vi "GeoData.vi"() -> ()   [LabVIEW 2017] (continued)
County\tH4\n6098\t9005\tWinsted\tCT\tLitchfield County\tH4\n6763\t9005\tMorris\tCT\tLitchfield County\tH4\n6779\t9005\tOakville\tCT\tLitchfield County\tH4\n6793\t9005\tWashington\tCT\tLitchfield County\tH4\n6786\t9005\tTerryville\tCT\tLitchfield County\tH4\n6782\t9005\tPlymouth\tCT\tLitchfield County\tH4\n6759\t9005\tLitchfield\tCT\tLitchfield County\tH4\n6753\t9005\tCornwall\tCT\tLitchfield County\tH4\n6708\t9005\tWaterbury\tCT\tLitchfield County\tH4\n6750\t9005\tBantam\tCT\tLitchfield County\tH4\n6756\t9005\tGoshen\tCT\tLitchfield County\tH4\n6757\t9005\tKent\tCT\tLitchfield County\tH4\n6068\t9005\tSalisbury\tCT\tLitchfield County\tH4\n6755\t9005\tGaylordsville\tCT\tLitchfield County\tH4\n6781\t9005\tPequabuck\tCT\tLitchfield County\tH4\n6792\t9005\tTorrington\tCT\tLitchfield County\tH4\n6031\t9005\tFalls village\tCT\tLitchfield County\tH4\n6069\t9005\tSharon\tCT\tLitchfield County\tH4\n6063\t9005\tBarkhamsted\tCT\tLitchfield County\tH4\n6751\t9005\tBethlehem\tCT\tLitchfield County\tH4\n6784\t9005\tSherman\tCT\tLitchfield County\tH4\n6791\t9005\tHarwinton\tCT\tLitchfield County\tH4\n6794\t9005\tWashington depot\tCT\tLitchfield County\tH4\n6804\t9005\tBrookfield\tCT\tLitchfield County\tH4\n6065\t9005\tRiverton\tCT\tLitchfield County\tH4\n6785\t9005\tSouth kent\tCT\tLitchfield County\tH4\n6783\t9005\tRoxbury\tCT\tLitchfield County\tH4\n6059\t9005\tNorth canton\tCT\tLitchfield County\tH4\n6010\t9005\tBristol\tCT\tLitchfield County\tH4\n6790\t9005\tTorrington\tCT\tLitchfield County\tH4\n6018\t9005\tCanaan\tCT\tLitchfield County\tH4\n6777\t9005\tNew preston marble dale\tCT\tLitchfield County\tH4\n6776\t9005\tNew milford\tCT\tLitchfield County\tH4\n6752\t9005\tBridgewater\tCT\tLitchfield County\tH4\n6796\t9005\tWest cornwall\tCT\tLitchfield County\tH4\n6079\t9005\tTaconic\tCT\tLitchfield County\tH4\n6024\t9005\tEast canaan\tCT\tLitchfield County\tH4\n6061\t9005\tPine meadow\tCT\tLitchfield County\tH4\n6039\t9005\tLakeville\tCT\tLitchfield County\tH4\n6058\t9005\tNorfolk\tCT\tLitchfield County\tH4\n6778\t9005\tNorthfield\tCT\tLitchfield County\tH4\n6798\t9005\tWoodbury\tCT\tLitchfield County\tH4\n6795\t9005\tWatertown\tCT\tLitchfield County\tH4\n6787\t9005\tThomaston\tCT\tLitchfield County\tH4\n6754\t9005\tCornwall bridge\tCT\tLitchfield County\tH4\n6758\t9005\tLakeside\tCT\tLitchfield County\tH4\n6073\t9007\tSouth glastonbury\tCT\tMiddlesex County\tH4\n6413\t9007\tClinton\tCT\tMiddlesex County\tH4\n6422\t9007\tDurham\tCT\tMiddlesex County\tH4\n6424\t9007\tEast hampton\tCT\tMiddlesex County\tH4\n6441\t9007\tHigganum\tCT\tMiddlesex County\tH4\n6420\t9007\tSalem\tCT\tMiddlesex County\tH4\n6442\t9007\tIvoryton\tCT\tMiddlesex County\tH4\n6456\t9007\tMiddle haddam\tCT\tMiddlesex County\tH4\n6426\t9007\tEssex\tCT\tMiddlesex County\tH4\n6475\t9007\tOld saybrook\tCT\tMiddlesex County\tH4\n6023\t9007\tEast berlin\tCT\tMiddlesex County\tH4\n6469\t9007\tMoodus\tCT\tMiddlesex County\tH4\n6480\t9007\tPortland\tCT\tMiddlesex County\tH4\n6414\t9007\tCobalt\tCT\tMiddlesex County\tH4\n6423\t9007\tEast haddam\tCT\tMiddlesex County\tH4\n6416\t9007\tCromwell\tCT\tMiddlesex County\tH4\n6409\t9007\tCenterbrook\tCT\tMiddlesex County\tH4\n6457\t9007\tMiddletown\tCT\tMiddlesex County\tH4\n6455\t9007\tMiddlefield\tCT\tMiddlesex County\tH4\n6459\t9007\tMiddletown\tCT\tMiddlesex County\tH4\n6412\t9007\tChester\tCT\tMiddlesex County\tH4\n6415\t9007\tColchester\tCT\tMiddlesex County\tH4\n6417\t9007\tDeep river\tCT\tMiddlesex County\tH4\n6419\t9007\tKillingworth\tCT\tMiddlesex County\tH4\n6438\t9007\tHaddam\tCT\tMiddlesex County\tH4\n6498\t9007\tWestbrook\tCT\tMiddlesex County\tH4\n6481\t9007\tRockfall\tCT\tMiddlesex County\tH4\n6422\t9009\tDurham\tCT\tNew Haven County\tH4\n6403\t9009\tBeacon falls\tCT\tNew Haven County\tH4\n6450\t9009\tMeriden\tCT\tNew Haven County\tH4\n6443\t9009\tMadison\tCT\tNew Haven County\tH4\n6483\t9009\tSeymour\tCT\tNew Haven County\tH4\n6770\t9009\tNaugatuck\tCT\tNew Haven County\tH4\n6779\t9009\tOakville\tCT\tNew Haven County\tH4\n6521\t9009\tNew haven\tCT\tNew Haven County\tH4\n6493\t9009\tWallingford\tCT\tNew Haven County\tH4\n6509\t9009\tNew haven\tCT\tNew Haven County\tH4\n6501\t9009\tNew haven\tCT\tNew Haven County\tH4\n6749\t9009\tWaterbury\tCT\tNew Haven County\tH4\n6703\t9009\tWaterbury\tCT\tNew Haven County\tH4\n6401\t9009\tAnsonia\tCT\tNew Haven County\tH4\n6461\t9009\tMilford\tCT\tNew Haven County\tH4\n6460\t9009\tMilford\tCT\tNew Haven County\tH4\n6489\t9009\tSouthington\tCT\tNew Haven County\tH4\n6511\t9009\tNew haven\tCT\tNew Haven County\tH4\n6720\t9009\tWaterbury\tCT\tNew Haven County\tH4\n6724\t9009\tWaterbury\tCT\tNew Haven County\tH4\n6533\t9009\tNew haven\tCT\tNew Haven County\tH4\n6488\t9009\tSouthbury\tCT\tNew Haven County\tH4\n6516\t9009\tWest haven\tCT\tNew Haven County\tH4\n6517\t9009\tHamden\tCT\tNew Haven County\tH4\n6518\t9009\tHamden\tCT\tNew Haven County\tH4\n6520\t9009\tNew haven\tCT\tNew Haven County\tH4\n6524\t9009\tBethany\tCT\tNew Haven County\tH4\n6708\t9009\tWaterbury\tCT\tNew Haven County\tH4\n6410\t9009\tCheshire\tCT\tNew Haven County\tH4\n6702\t9009\tWaterbury\tCT\tNew Haven County\tH4\n6532\t9009\tNew haven\tCT\tNew Haven County\tH4\n6505\t9009\tNew haven\tCT\tNew Haven County\tH4\n6507\t9009\tNew haven\tCT\tNew Haven County\tH4\n6411\t9009\tCheshire\tCT\tNew Haven County\tH4\n6037\t9009\tBerlin\tCT\tNew Haven County\tH4\n6418\t9009\tDerby\tCT\tNew Haven County\tH4\n6451\t9009\tMeriden\tCT\tNew Haven County\tH4\n6473\t9009\tNorth haven\tCT\tNew Haven County\tH4\n6477\t9009\tOrange\tCT\tNew Haven County\tH4\n6514\t9009\tHamden\tCT\tNew Haven County\tH4\n6510\t9009\tNew haven\tCT\tNew Haven County\tH4\n6515\t9009\tNew haven\tCT\tNew Haven County\tH4\n6762\t9009\tMiddlebury\tCT\tNew Haven County\tH4\n6487\t9009\tSouth britain\tCT\tNew Haven County\tH4\n6723\t9009\tWaterbury\tCT\tNew Haven County\tH4\n6701\t9009\tWaterbury\tCT\tNew Haven County\tH4\n6530\t9009\tNew haven\tCT\tNew Haven County\tH4\n6495\t9009\tWallingford\tCT\tNew Haven County\tH4\n6504\t9009\tNew haven\tCT\tNew Haven County\tH4\n6535\t9009\tNew haven\tCT\tNew Haven County\tH4\n6536\t9009\tNew haven\tCT\tNew Haven County\tH4\n6437\t9009\tGuilford\tCT\tNew Haven County\tH4\n6492\t9009\tWallingford\tCT\tNew Haven County\tH4\n6479\t9009\tPlantsville\tCT\tNew Haven County\tH4\n6471\t9009\tNorth branford\tCT\tNew Haven County\tH4\n6525\t9009\tWoodbridge\tCT\tNew Haven County\tH4\n6706\t9009\tWaterbury\tCT\tNew Haven County\tH4\n6712\t9009\tProspect\tCT\tNew Haven County\tH4\n6506\t9009\tNew haven\tCT\tNew Haven County\tH4\n6502\t9009\tNew haven\tCT\tNew Haven County\tH4\n6534\t9009\tNew haven\tCT\tNew Haven County\tH4\n6537\t9009\tNew haven\tCT\tNew Haven County\tH4\n6472\t9009\tNorthford\tCT\tNew Haven County\tH4\n6519\t9009\tNew haven\tCT\tNew Haven County\tH4\n6705\t9009\tWaterbury\tCT\tNew Haven County\tH4\n6716\t9009\tWolcott\tCT\tNew Haven County\tH4\n6710\t9009\tWaterbury\tCT\tNew Haven County\tH4\n6503\t9009\tNew haven\tCT\tNew Haven County\tH4\n6721\t9009\tWaterbury\tCT\tNew Haven County\tH4\n6508\t9009\tNew haven\tCT\tNew Haven County\tH4\n6540\t9009\tNew haven\tCT\tNew Haven County\tH4\n6494\t9009\tWallingford\tCT\tNew Haven County\tH4\n6405\t9009\tBranford\tCT\tNew Haven County\tH4\n6478\t9009\tOxford\tCT\tNew Haven County\tH4\n6513\t9009\tNew haven\tCT\tNew Haven County\tH4\n6512\t9009\tEast haven\tCT\tNew Haven County\tH4\n6704\t9009\tWaterbury\tCT\tNew Haven County\tH4\n6722\t9009\tWaterbury\tCT\tNew Haven County\tH4\n6538\t9009\tNew haven\tCT\tNew Haven County\tH4\n6531\t9009\tNew haven\tCT\tNew Haven County\tH4\n6408\t9009\tCheshire\tCT\tNew Haven County\tH4\n6231\t9011\tAmston\tCT\tNew London County\tH4\n6339\t9011\tLedyard\tCT\tNew London County\tH4\n6359\t9011\tNorth stonington\tCT\tNew London County\tH4\n6374\t9011\tPlainfield\tCT\tNew London County\tH4\n6383\t9011\tVersailles\tCT\tNew London County\tH4\n6372\t9011\tOld mystic\tCT\tNew London County\tH4\n6330\t9011\tBaltic\tCT\tNew London County\tH4\n6385\t9011\tWaterford\tCT\tNew London County\tH4\n6420\t9011\tSalem\tCT\tNew London County\tH4\n6384\t9011\tVoluntown\tCT\tNew London County\tH4\n6380\t9011\tTaftville\tCT\tNew London County\tH4\n6336\t9011\tGilman\tCT\tNew London County\tH4\n6439\t9011\tHadlyme\tCT\tNew London County\tH4\n6335\t9011\tGales ferry\tCT\tNew London County\tH4\n6351\t9011\tJewett city\tCT\tNew London County\tH4\n6375\t9011\tQuaker hill\tCT\tNew London County\tH4\n6382\t9011\tUncasville\tCT\tNew London County\tH4\n6379\t9011\tPawcatuck\tCT\tNew London County\tH4\n6360\t9011\tNorwich\tCT\tNew London County\tH4\n6254\t9011\tNorth franklin\tCT\tNew London County\tH4\n6349\t9011\tGroton\tCT\tNew London County\tH4\n6357\t9011\tNiantic\tCT\tNew London County\tH4\n6370\t9011\tOakdale\tCT\tNew London County\tH4\n6389\t9011\tYantic\tCT\tNew London County\tH4\n6388\t9011\tWest mystic\tCT\tNew London County\tH4\n6371\t9011\tOld lyme\tCT\tNew London County\tH4\n6333\t9011\tEast lyme\tCT\tNew London County\tH4\n6334\t9011\tBozrah\tCT\tNew London County\tH4\n6415\t9011\tColchester\tCT\tNew London County\tH4\n6350\t9011\tHanover\tCT\tNew London County\tH4\n6338\t9011\tMashantucket\tCT\tNew London County\tH4\n6353\t9011\tMontville\tCT\tNew London County\tH4\n6249\t9011\tLebanon\tCT\tNew London County\tH4\n6340\t9011\tGroton\tCT\tNew London County\tH4\n6355\t9011\tMystic\tCT\tNew London County\tH4\n6320\t9011\tNew london\tCT\tNew London County\tH4\n6378\t9011\tStonington\tCT\tNew London County\tH4\n6365\t9011\tPreston\tCT\tNew London County\tH4\n6376\t9011\tSouth lyme\tCT\tNew London County\tH4\n6066\t9013\tVernon rockville\tCT\tTolland County\tH4\n6076\t9013\tStafford springs\tCT\tTolland County\tH4\n6231\t9013\tAmston\tCT\tTolland County\tH4\n6072\t9013\tSomersville\tCT\tTolland County\tH4\n6077\t9013\tStaffordville\tCT\tTolland County\tH4\n6232\t9013\tAndover\tCT\tTolland County\tH4\n6242\t9013\tEastford\tCT\tTolland County\tH4\n6238\t9013\tCoventry\tCT\tTolland County\tH4\n6269\t9013\tStorrs mansfield\tCT\tTolland County\tH4\n6251\t9013\tMansfield depot\tCT\tTolland County\tH4\n6084\t9013\tTolland\tCT\tTolland County\tH4\n6074\t9013\tSouth windsor\tCT\tTolland County\tH4\n6237\t9013\tColumbia\tCT\tTolland County\tH4\n6033\t9013\tGlastonbury\tCT\tTolland County\tH4\n6042\t9013\tManchester\tCT\tTolland County\tH4\n6043\t9013\tBolton\tCT\tTolland County\tH4\n6071\t9013\tSomers\tCT\tTolland County\tH4\n6226\t9013\tWillimantic\tCT\tTolland County\tH4\n6268\t9013\tStorrs mansfield\tCT\tTolland County\tH4\n6279\t9013\tWillington\tCT\tTolland County\tH4\n6235\t9013\tChaplin\tCT\tTolland County\tH4\n6250\t9013\tMansfield center\tCT\tTolland County\tH4\n6415\t9013\tColchester\tCT\tTolland County\tH4\n6029\t9013\tEllington\tCT\tTolland County\tH4\n6248\t9013\tHebron\tCT\tTolland County\tH4\n6447\t9013\tMarlborough\tCT\tTolland County\tH4\n6075\t9013\tStafford\tCT\tTolland County\tH4\n6277\t9015\tThompson\tCT\tWindham County\tH4\n6374\t9015\tPlainfield\tCT\tWindham County\tH4\n6282\t9015\tWoodstock valley\tCT\tWindham County\tH4\n6266\t9015\tSouth windham\tCT\tWindham County\tH4\n6280\t9015\tWindham\tCT\tWindham County\tH4\n6246\t9015\tGrosvenor dale\tCT\tWindham County\tH4\n6234\t9015\tBrooklyn\tCT\tWindham County\tH4\n6330\t9015\tBaltic\tCT\tWindham County\tH4\n6384\t9015\tVoluntown\tCT\tWindham County\tH4\n6255\t9015\tNorth grosvenordale\tCT\tWindham County\tH4\n6242\t9015\tEastford\tCT\tWindham County\tH4\n6373\t9015\tOneco\tCT\tWindham County\tH4\n6239\t9015\tDanielson\tCT\tWindham County\tH4\n6259\t9015\tPomfret center\tCT\tWindham County\tH4\n6247\t9015\tHampton\tCT\tWindham County\tH4\n6260\t9015\tPutnam\tCT\tWindham County\tH4\n6281\t9015\tWoodstock\tCT\tWindham County\tH4\n6351\t9015\tJewett city\tCT\tWindham County\tH4\n6377\t9015\tSterling\tCT\tWindham County\tH4\n6263\t9015\tRogers\tCT\tWindham County\tH4\n6230\t9015\tAbington\tCT\tWindham County\tH4\n6331\t9015\tCanterbury\tCT\tWindham County\tH4\n6354\t9015\tMoosup\tCT\tWindham County\tH4\n6332\t9015\tCentral village\tCT\tWindham County\tH4\n6256\t9015\tNorth windham\tCT\tWindham County\tH4\n6226\t9015\tWillimantic\tCT\tWindham County\tH4\n6279\t9015\tWillington\tCT\tWindham County\tH4\n6244\t9015\tEast woodstock\tCT\tWindham County\tH4\n6262\t9015\tQuinebaug\tCT\tWindham County\tH4\n6264\t9015\tScotland\tCT\tWindham County\tH4\n6241\t9015\tDayville\tCT\tWindham County\tH4\n6235\t9015\tChaplin\tCT\tWindham County\tH4\n6250\t9015\tMansfield center\tCT\tWindham County\tH4\n6258\t9015\tPomfret\tCT\tWindham County\tH4\n6267\t9015\tSouth woodstock\tCT\tWindham County\tH4\n6278\t9015\tAshford\tCT\tWindham County\tH4\n6387\t9015\tWauregan\tCT\tWindham County\tH4\n6243\t9015\tEast killingly\tCT\tWindham County\tH4\n6233\t9015\tBallouville\tCT\tWindham County\tH4\n19977\t10001\tSmyrna\tDE\tKent County\tH1\n19903\t10001\tDover\tDE\tKent County\tH1\n19955\t10001\tKenton\tDE\tKent County\tH1\n19902\t10001\tDover afb\tDE\tKent County\tH1\n19934\t10001\tCamden wyoming\tDE\tKent County\tH1\n19946\t10001\tFrederica\tDE\tKent County\tH1\n19950\t10001\tGreenwood\tDE\tKent County\tH1\n19936\t10001\tCheswold\tDE\tKent County\tH1\n19901\t10001\tDover\tDE\tKent County\tH1\n19952\t10001\tHarrington\tDE\tKent County\tH1\n19938\t10001\tClayton\tDE\tKent County\tH1\n19953\t10001\tHartly\tDE\tKent County\tH1\n19962\t10001\tMagnolia\tDE\tKent County\tH1\n19954\t10001\tHouston\tDE\tKent County\tH1\n19904\t10001\tDover\tDE\tKent County\tH1\n19963\t10001\tMilford\tDE\tKent County\tH1\n19980\t10001\tWoodside\tDE\tKent County\tH1\n19943\t10001\tFelton\tDE\tKent County\tH1\n19964\t10001\tMarydel\tDE\tKent County\tH1\n19979\t10001\tViola\tDE\tKent County\tH1\n19961\t10001\tLittle creek\tDE\tKent County\tH1\n19711\t10003\tNewark\tDE\tNew Castle County\tH1\n19977\t10003\tSmyrna\tDE\tNew Castle County\tH1\n19716\t10003\tNewark\tDE\tNew Castle County\tH1\n19718\t10003\tNewark\tDE\tNew Castle County\tH1\n19708\t10003\tKirkwood\tDE\tNew Castle County\tH1\n19702\t10003\tNewark\tDE\tNew Castle County\tH1\n19713\t10003\tNewark\tDE\tNew Castle County\tH1\n19720\t10003\tNew castle\tDE\tNew Castle County\tH1\n19802\t10003\tWilmington\tDE\tNew Castle County\tH1\n19717\t10003\tNewark\tDE\tNew Castle County\tH1\n19899\t10003\tWilmington\tDE\tNew Castle County\tH1\n19892\t10003\tWilmington\tDE\tNew Castle County\tH1\n19701\t10003\tBear\tDE\tNew Castle County\tH1\n19712\t10003\tNewark\tDE\tNew Castle County\tH1\n19710\t10003\tMontchanin\tDE\tNew Castle County\tH1\n19807\t10003\tWilmington\tDE\tNew Castle County\tH1\n19732\t10003\tRockland\tDE\tNew Castle County\tH1\n19726\t10003\tNew castle\tDE\tNew Castle County\tH1\n19736\t10003\tYorklyn\tDE\tNew Castle County\tH1\n19707\t10003\tHockessin\tDE\tNew Castle County\tH1\n19734\t10003\tTownsend\tDE\tNew Castle County\tH1\n19730\t10003\tOdessa\tDE\tNew Castle County\tH1\n19808\t10003\tWilmington\tDE\tNew Castle County\tH1\n19938\t10003\tClayton\tDE\tNew Castle County\tH1\n19890\t10003\tWilmington\tDE\tNew Castle County\tH1\n19898\t10003\tWilmington\tDE\tNew Castle County\tH1\n19721\t10003\tNew castle\tDE\tNew Castle County\tH1\n19703\t10003\tClaymont\tDE\tNew Castle County\tH1\n19715\t10003\tNewark\tDE\tNew Castle County\tH1\n19731\t10003\tPort penn\tDE\tNew Castle County\tH1\n19897\t10003\tWilmington\tDE\tNew Castle County\tH1\n19706\t10003\tDelaware city\tDE\tNew Castle County\tH1\n19709\t10003\tMiddletown\tDE\tNew Castle County\tH1\n19803\t10003\tWilmington\tDE\tNew Castle County\tH1\n19810\t10003\tWilmington\tDE\tNew Castle County\tH1\n19735\t10003\tWinterthur\tDE\tNew Castle County\tH1\n19714\t10003\tNewark\tDE\tNew Castle County\tH1\n19884\t10003\tWilmington\tDE\tNew Castle County\tH1\n19894\t10003\tWilmington\tDE\tNew Castle County\tH1\n19896\t10003\tWilmington\tDE\tNew Castle County\tH1\n19804\t10003\tWilmington\tDE\tNew Castle County\tH1\n19801\t10003\tWilmington\tDE\tNew Castle County\tH1\n19806\t10003\tWilmington\tDE\tNew Castle County\tH1\n19733\t10003\tSaint georges\tDE\tNew Castle County\tH1\n19895\t10003\tWilmington\tDE\tNew Castle County\tH1\n19805\t10003\tWilmington\tDE\tNew Castle County\tH1\n19809\t10003\tWilmington\tDE\tNew Castle County\tH1\n19958\t10005\tLewes\tDE\tSussex County\tH1\n19939\t10005\tDagsboro\tDE\tSussex County\tH1\n19956\t10005\tLaurel\tDE\tSussex County\tH1\n19967\t10005\tMillville\tDE\tSussex County\tH1\n19950\t10005\tGreenwood\tDE\tSussex County\tH1\n19944\t10005\tFenwick island\tDE\tSussex County\tH1\n19940\t10005\tDelmar\tDE\tSussex County\tH1\n19968\t10005\tMilton\tDE\tSussex County\tH1\n19952\t10005\tHarrington\tDE\tSussex County\tH1\n19941\t10005\tEllendale\tDE\tSussex County\tH1\n19931\t10005\tBethel\tDE\tSussex County\tH1\n19945\t10005\tFrankford\tDE\tSussex County\tH1\n19951\t10005\tHarbeson\tDE\tSussex County\tH1\n19973\t10005\tSeaford\tDE\tSussex County\tH1\n19947\t10005\tGeorgetown\tDE\tSussex County\tH1\n19971\t10005\tRehoboth beach\tDE\tSussex County\tH1\n19966\t10005\tMillsboro\tDE\tSussex County\tH1\n19975\t10005\tSelbyville\tDE\tSussex County\tH1\n19930\t10005\tBethany beach\tDE\tSussex County\tH1\n19963\t10005\tMilford\tDE\tSussex County\tH1\n19970\t10005\tOcean view\tDE\tSussex County\tH1\n19933\t10005\tBridgeville\tDE\tSussex County\tH1\n19960\t10005\tLincoln\tDE\tSussex County\tH1\n19969\t10005\tNassau\tDE\tSussex County\tH1\n20001\t11001\tWashington\tDC\tDistrict of Columbia\tH6\n20005\t11001\tWashington\tDC\tDistrict of Columbia\tH6\n20017\t11001\tWashington\tDC\tDistrict of Columbia\tH6\n20374\t11001\tWashington navy yard\tDC\tDistrict of Columbia\tH6\n20254\t11001\tWashington\tDC\tDistrict of Columbia\tH6\n20426\t11001\tWashington\tDC\tDistrict of Columbia\tH6\n20544\t11001\tWashington\tDC\tDistrict of Columbia\tH6\n20063\t11001\tWashington\tDC\tDistrict of Columbia\tH6\n20557\t11001\tWashington\tDC\tDistrict of Columbia\tH6\n20441\t11001\tWashington\tDC\tDistrict of Columbia\tH6\n20534\t11001\tWashington\tDC\tDistrict of Columbia\tH6\n20217\t11001\tWashington\tDC\tDistrict of Columbia\tH6\n20391\t11001\tWashington navy yard\tDC\tDistrict of Columbia\tH6\n20507\t11001\tWashington\tDC\tDistrict of Columbia\tH6\n20591\t11001\tWashington\tDC\tDistrict of Columbia\tH6\n20245\t11001\tWashington\tDC\tDistrict of Columbia\tH6\n20303\t11001\tWashington\tDC\tDistrict of Columbia\tH6\n20204\t11001\tWashington\tDC\tDistrict of Columbia\tH6\n20405\t11001\tWashington\tDC\tDistrict of Columbia\tH6\n20542\t11001\tWashington\tDC\tDistrict of Columbia\tH6\n20573\t11001\tWashington\tDC\tDistrict of Columbia\tH6\n20235\t11001\tWashington\tDC\tDistrict of Columbia\tH6\n56998\t11001\tParcel return service\tDC\tDistrict of Columbia\tH6\n20004\t11001\tWashington\tDC\tDistrict of Columbia\tH6\n20528\t11001\tWashington\tDC\tDistrict of Columbia\tH6\n20038\t11001\tWashington\tDC\tDistrict of Columbia\tH6\n20372\t11001\tWashington\tDC\tDistrict of Columbia\tH6\n20520\t11001\tWashington\tDC\tDistrict of Columbia\tH6\n20027\t11001\tWashington\tDC\tDistrict of Columbia\tH6\n20039\t11001\tWashington\tDC\tDistrict of Columbia\tH6\n20056\t11001\tWashington\tDC\tDistrict of Columbia\tH6\n20220\t11001\tWashington\tDC\tDistrict of Columbia\tH6\n20066\t11001\tWashington\tDC\tDistrict of Columbia\tH6\n20057\t11001\tWashington\tDC\tDistrict of Columbia\tH6\n20500\t11001\tWashington\tDC\tDistrict of Columbia\tH6\n20380\t11001\tWashington\tDC\tDistrict of Columbia\tH6\n20575\t11001\tWashington\tDC\tDistrict of Columbia\tH6\n20560\t11001\tWashington\tDC\tDistrict of Columbia\tH6\n20431\t11001\tWashington\tDC\tDistrict of Columbia\tH6\n20463\t11001\tWashington\tDC\tDistrict of Columbia\tH6\n20506\t11001\tWashington\tDC\tDistrict of Columbia\tH6\n20062\t11001\tWashington\tDC\tDistrict of Columbia\tH6\n20268\t11001\tWashington\tDC\tDistrict of Columbia\tH6\n20504\t11001\tWashington\tDC\tDistrict of Columbia\tH6\n20521\t11001\tWashington\tDC\tDistrict of Columbia\tH6\n20003\t11001\tWashington\tDC\tDistrict of Columbia\tH6\n20008\t11001\tWashington\tDC\tDistrict of Columbia\tH6\n20015\t11001\tWashington\tDC\tDistrict of Columbia\tH6\n20035\t11001\tWashington\tDC\tDistrict of Columbia\tH6\n20029\t11001\tWashington\tDC\tDistrict of Columbia\tH6\n20472\t11001\tWashington\tDC\tDistrict of Columbia\tH6\n20529\t11001\tWashington\tDC\tDistrict of Columbia\tH6\n20404\t11001\tWashington\tDC\tDistrict of Columbia\tH6\n20052\t11001\tWashington\tDC\tDistrict of Columbia\tH6\n20059\t11001\tWashington\tDC\tDistrict of Columbia\tH6\n20045\t11001\tWashington\tDC\tDistrict of Columbia\tH6\n20319\t11001\tWashington\tDC\tDistrict of Columbia\tH6\n20566\t11001\tWashington\tDC\tDistrict of Columbia\tH6\n20541\t11001\tWashington\tDC\tDistrict of Columbia\tH6\n20239\t11001\tWashington\tDC\tDistrict of Columbia\tH6\n20411\t11001\tWashington\tDC\tDistrict of Columbia\tH6\n20228\t11001\tWashington\tDC\tDistrict of Columbia\tH6\n20524\t11001\tWashington\tDC\tDistrict of Columbia\tH6\n20270\t11001\tWashington\tDC\tDistrict of Columbia\tH6\n20433\t11001\tWashington\tDC\tDistrict of Columbia\tH6\n20424\t11001\tWashington\tDC\tDistrict of Columbia\tH6\n20422\t11001\tWashington\tDC\tDistrict of Columbia\tH6\n20535\t11001\tWashington\tDC\tDistrict of Columbia\tH6\n20436\t11001\tWashington\tDC\tDistrict of Columbia\tH6\n20538\t11001\tWashington\tDC\tDistrict of Columbia\tH6\n20071\t11001\tWashington\tDC\tDistrict of Columbia\tH6\n20237\t11001\tWashington\tDC\tDistrict of Columbia\tH6\n20546\t11001\tWashington\tDC\tDistrict of Columbia\tH6\n20047\t11001\tWashington\tDC\tDistrict of Columbia\tH6\n20410\t11001\tWashington\tDC\tDistrict of Columbia\tH6\n20439\t11001\tWashington\tDC\tDistrict of Columbia\tH6\n20016\t11001\tWashington\tDC\tDistrict of Columbia\tH6\n20024\t11001\tWashington\tDC\tDistrict of Columbia\tH6\n20036\t11001\tWashington\tDC\tDistrict of Columbia\tH6\n20376\t11001\tWashington navy yard\tDC\tDistrict of Columbia\tH6\n20536\t11001\tWashington\tDC\tDistrict of Columbia\tH6\n20013\t11001\tWashington\tDC\tDistrict of Columbia\tH6\n20437\t11001\tWashington\tDC\tDistrict of Columbia\tH6\n20202\t11001\tWashington\tDC\tDistrict of Columbia\tH6\n20549\t11001\tWashington\tDC\tDistrict of Columbia\tH6\n20033\t11001\tWashington\tDC\tDistrict of Columbia\tH6\n20201\t11001\tWashington\tDC\tDistrict of Columbia\tH6\n20211\t11001\tWashington\tDC\tDistrict of Columbia\tH6\n20055\t11001\tWashington\tDC\tDistrict of Columbia\tH6\n20447\t11001\tWashington\tDC\tDistrict of Columbia\tH6\n20460\t11001\tWashington\tDC\tDistrict of Columbia\tH6\n20442\t11001\tWashington\tDC\tDistrict of Columbia\tH6\n20590\t11001\tWashington\tDC\tDistrict of Columbia\tH6\n20526\t11001\tWashington\tDC\tDistrict of Columbia\tH6\n20398\t11001\tWashington navy yard\tDC\tDistrict of Columbia\tH6\n20565\t11001\tWashington\tDC\tDistrict of Columbia\tH6\n20418\t11001\tWashington\tDC\tDistrict of Columbia\tH6\n20456\t11001\tWashington\tDC\tDistrict of Columbia\tH6\n20539\t11001\tWashington\tDC\tDistrict of Columbia\tH6\n20435\t11001\tWashington\tDC\tDistrict of Columbia\tH6\n20451\t11001\tWashington\tDC\tDistrict of Columbia\tH6\n20415\t11001\tWashington\tDC\tDistrict of Columbia\tH6\n20417\t11001\tWashington\tDC\tDistrict of Columbia\tH6\n20002\t11001\tWashington\tDC\tDistrict of Columbia\tH6\n20007\t11001\tWashington\tDC\tDistrict of Columbia\tH6\n20011\t11001\tWashington\tDC\tDistrict of Columbia\tH6\n20018\t11001\tWashington\tDC\tDistrict of Columbia\tH6\n20091\t11001\tWashington\tDC\tDistrict of Columbia\tH6\n20530\t11001\tWashington\tDC\tDistrict of Columbia\tH6\n20026\t11001\tWashington\tDC\tDistrict of Columbia\tH6\n20429\t11001\tWashington\tDC\tDistrict of Columbia\tH6\n20402\t11001\tWashington\tDC\tDistrict of Columbia\tH6\n20226\t11001\tWashington\tDC\tDistrict of Columbia\tH6\n20509\t11001\tWashington\tDC\tDistrict of Columbia\tH6\n20594\t11001\tWashington\tDC\tDistrict of Columbia\tH6\n20414\t11001\tWashington\tDC\tDistrict of Columbia\tH6\n20505\t11001\tWashington\tDC\tDistrict of Columbia\tH6\n20064\t11001\tWashington\tDC\tDistrict of Columbia\tH6\n20219\t11001\tWashington\tDC\tDistrict of Columbia\tH6\n20241\t11001\tWashington\tDC\tDistrict of Columbia\tH6\n20289\t11001\tWashington\tDC\tDistrict of Columbia\tH6\n20049\t11001\tWashington\tDC\tDistrict of Columbia\tH6\n20212\t11001\tWashington\tDC\tDistrict of Columbia\tH6\n20240\t11001\tWashington\tDC\tDistrict of Columbia\tH6\n20042\t11001\tWashington\tDC\tDistrict of Columbia\tH6\n20218\t11001\tWashington\tDC\tDistrict of Columbia\tH6\n20586\t11001\tWashington\tDC\tDistrict of Columbia\tH6\n20444\t11001\tWashington\tDC\tDistrict of Columbia\tH6\n20554\t11001\tWashington\tDC\tDistrict of Columbia\tH6\n20390\t11001\tWashington\tDC\tDistrict of Columbia\tH6\n20533\t11001\tWashington\tDC\tDistrict of Columbia\tH6\n20552\t11001\tWashington\tDC\tDistrict of Columbia\tH6\n20423\t11001\tWashington\tDC\tDistrict of Columbia\tH6\n20037\t11001\tWashington\tDC\tDistrict of Columbia\tH6\n20421\t11001\tWashington\tDC\tDistrict of Columbia\tH6\n20250\t11001\tWashington\tDC\tDistrict of Columbia\tH6\n20373\t11001\tNaval anacost annex\tDC\tDistrict of Columbia\tH6\n20510\t11001\tWashington\tDC\tDistrict of Columbia\tH6\n20044\t11001\tWashington\tDC\tDistrict of Columbia\tH6\n20577\t11001\tWashington\tDC\tDistrict of Columbia\tH6\n20318\t11001\tWashington\tDC\tDistrict of Columbia\tH6\n20229\t11001\tWashington\tDC\tDistrict of Columbia\tH6\n20401\t11001\tWashington\tDC\tDistrict of Columbia\tH6\n20571\t11001\tWashington\tDC\tDistrict of Columbia\tH6\n20597\t11001\tWashington\tDC\tDistrict of Columbia\tH6\n20523\t11001\tWashington\tDC\tDistrict of Columbia\tH6\n20503\t11001\tWashington\tDC\tDistrict of Columbia\tH6\n20434\t11001\tWashington\tDC\tDistrict of Columbia\tH6\n20580\t11001\tWashington\tDC\tDistrict of Columbia\tH6\n20073\t11001\tWashington\tDC\tDistrict of Columbia\tH6\n20508\t11001\tWashington\tDC\tDistrict of Columbia\tH6\n20306\t11001\tWashington\tDC\tDistrict of Columbia\tH6\n20230\t11001\tWashington\tDC\tDistrict of Columbia\tH6\n20227\t11001\tWashington\tDC\tDistrict of Columbia\tH6\n20340\t11001\tWashington\tDC\tDistrict of Columbia\tH6\n20419\t11001\tWashington\tDC\tDistrict of Columbia\tH6\n20543\t11001\tWashington\tDC\tDistrict of Columbia\tH6\n20547\t11001\tWashington\tDC\tDistrict of Columbia\tH6\n20210\t11001\tWashington\tDC\tDistrict of Columbia\tH6\n20440\t11001\tWashington\tDC\tDistrict of Columbia\tH6\n20222\t11001\tWashington\tDC\tDistrict of Columbia\tH6\n20053\t11001\tWashington\tDC\tDistrict of Columbia\tH6\n20581\t11001\tWashington\tDC\tDistrict of Columbia\tH6\n20555\t11001\tWashington\tDC\tDistrict of Columbia\tH6\n20006\t11001\tWashington\tDC\tDistrict of Columbia\tH6\n20010\t11001\tWashington\tDC\tDistrict of Columbia\tH6\n20012\t11001\tWashington\tDC\tDistrict of Columbia\tH6\n20019\t11001\tWashington\tDC\tDistrict of Columbia\tH6\n20020\t11001\tWashington\tDC\tDistrict of Columbia\tH6\n20427\t11001\tWashington\tDC\tDistrict of Columbia\tH6\n20515\t11001\tWashington\tDC\tDistrict of Columbia\tH6\n20522\t11001\tWashington\tDC\tDistrict of Columbia\tH6\n20221\t11001\tWashington\tDC\tDistrict of Columbia\tH6\n20559\t11001\tWashington\tDC\tDistrict of Columbia\tH6\n20043\t11001\tWashington\tDC\tDistrict of Columbia\tH6\n20428\t11001\tWashington\tDC\tDistrict of Columbia\tH6\n20593\t11001\tWashington\tDC\tDistrict of Columbia\tH6\n20375\t11001\tWashington\tDC\tDistrict of Columbia\tH6\n20242\t11001\tWashington\tDC\tDistrict of Columbia\tH6\n20570\t11001\tWashington\tDC\tDistrict of Columbia\tH6\n20203\t11001\tWashington\tDC\tDistrict of Columbia\tH6\n20370\t11001\tWashington\tDC\tDistrict of Columbia\tH6\n20223\t11001\tWashington\tDC\tDistrict of Columbia\tH6\n20425\t11001\tWashington\tDC\tDistrict of Columbia\tH6\n20525\t11001\tWashington\tDC\tDistrict of Columbia\tH6\n20260\t11001\tWashington\tDC\tDistrict of Columbia\tH6\n20413\t11001\tWashington\tDC\tDistrict of Columbia\tH6\n20576\t11001\tWashington\tDC\tDistrict of Columbia\tH6\n20076\t11001\tWashington\tDC\tDistrict of Columbia\tH6\n20572\t11001\tWashington\tDC\tDistrict of Columbia\tH6\n20208\t11001\tWashington\tDC\tDistrict of Columbia\tH6\n20244\t11001\tWashington\tDC\tDistrict of Columbia\tH6\n20407\t11001\tWashington\tDC\tDistrict of Columbia\tH6\n20551\t11001\tWashington\tDC\tDistrict of Columbia\tH6\n20408\t11001\tWashington\tDC\tDistrict of Columbia\tH6\n20009\t11001\tWashington\tDC\tDistrict of Columbia\tH6\n20032\t11001\tWashington\tDC\tDistrict of Columbia\tH6\n20040\t11001\tWashington\tDC\tDistrict of Columbia\tH6\n20090\t11001\tWashington\tDC\tDistrict of Columbia\tH6\n20540\t11001\tWashington\tDC\tDistrict of Columbia\tH6\n20030\t11001\tWashington\tDC\tDistrict of Columbia\tH6\n20585\t11001\tWashington\tDC\tDistrict of Columbia\tH6\n20215\t11001\tWashington\tDC\tDistrict of Columbia\tH6\n20416\t11001\tWashington\tDC\tDistrict of Columbia\tH6\n20060\t11001\tWashington\tDC\tDistrict of Columbia\tH6\n20392\t11001\tWashington\tDC\tDistrict of Columbia\tH6\n20553\t11001\tWashington\tDC\tDistrict of Columbia\tH6\n20065\t11001\tWashington\tDC\tDistrict of Columbia\tH6\n20216\t11001\tWashington\tDC\tDistrict of Columbia\tH6\n20579\t11001\tWashington\tDC\tDistrict of Columbia\tH6\n20388\t11001\tWashington navy yard\tDC\tDistrict of Columbia\tH6\n20531\t11001\tWashington\tDC\tDistrict of Columbia\tH6\n20412\t11001\tWashington\tDC\tDistrict of Columbia\tH6\n20527\t11001\tWashington\tDC\tDistrict of Columbia\tH6\n20548\t11001\tWashington\tDC\tDistrict of Columbia\tH6\n20403\t11001\tWashington\tDC\tDistrict of Columbia\tH6\n20224\t11001\tWashington\tDC\tDistrict of Columbia\tH6\n20213\t11001\tWashington\tDC\tDistrict of Columbia\tH6\n20420\t11001\tWashington\tDC\tDistrict of Columbia\tH6\n32601\t12001\tGainesville\tFL\tAlachua County\tH1\n32605\t12001\tGainesville\tFL\tAlachua County\tH1\n32635\t12001\tGainesville\tFL\tAlachua County\tH1\n32612\t12001\tGainesville\tFL\tAlachua County\tH1\n32608\t12001\tGainesville\tFL\tAlachua County\tH1\n32609\t12001\tGainesville\tFL\tAlachua County\tH1\n32614\t12001\tGainesville\tFL\tAlachua County\tH1\n32641\t12001\tGainesville\tFL\tAlachua County\tH1\n32640\t12001\tHawthorne\tFL\tAlachua County\tH1\n32631\t12001\tEarleton\tFL\tAlachua County\tH1\n32633\t12001\tEvinston\tFL\tAlachua County\tH1\n32662\t12001\tLochloosa\tFL\tAlachua County\tH1\n32667\t12001\tMicanopy\tFL\tAlachua County\tH1\n32669\t12001\tNewberry\tFL\tAlachua County\tH1\n32627\t12001\tGainesville\tFL\tAlachua County\tH1\n32610\t12001\tGainesville\tFL\tAlachua County\tH1\n32606\t12001\tGainesville\tFL\tAlachua County\tH1\n32622\t12001\tBrooker\tFL\tAlachua County\tH1\n32666\t12001\tMelrose\tFL\tAlachua County\tH1\n32654\t12001\tIsland grove\tFL\tAlachua County\tH1\n32618\t12001\tArcher\tFL\tAlachua County\tH1\n32696\t12001\tWilliston\tFL\tAlachua County\tH1\n32044\t12001\tHampton\tFL\tAlachua County\tH1\n32604\t12001\tGainesville\tFL\tAlachua County\tH1\n32611\t12001\tGainesville\tFL\tAlachua County\tH1\n32607\t12001\tGainesville\tFL\tAlachua County\tH1\n32643\t12001\tHigh springs\tFL\tAlachua County\tH1\n32603\t12001\tGainesville\tFL\tAlachua County\tH1\n32615\t12001\tAlachua\tFL\tAlachua County\tH1\n32653\t12001\tGainesville\tFL\tAlachua County\tH1\n32694\t12001\tWaldo\tFL\tAlachua County\tH1\n32658\t12001\tLa crosse\tFL\tAlachua County\tH1\n32234\t12003\tJacksonville\tFL\tBaker County\tH1\n32040\t12003\tGlen saint mary\tFL\tBaker County\tH1\n32087\t12003\tSanderson\tFL\tBaker County\tH1\n32063\t12003\tMacclenny\tFL\tBaker County\tH1\n32405\t12005\tPanama city\tFL\tBay County\tH1\n32403\t12005\tPanama city\tFL\tBay County\tH1\n32417\t12005\tPanama city\tFL\tBay County\tH1\n32409\t12005\tPanama city\tFL\tBay County\tH1\n32406\t12005\tPanama city\tFL\tBay County\tH1\n32428\t12005\tChipley\tFL\tBay County\tH1\n32456\t12005\tPort saint joe\tFL\tBay County\tH1\n32437\t12005\tEbro\tFL\tBay County\tH1\n32411\t12005\tPanama city\tFL\tBay County\tH1\n32438\t12005\tFountain\tFL\tBay County\tH1\n32465\t12005\tWewahitchka\tFL\tBay County\tH1\n32408\t12005\tPanama city\tFL\tBay County\tH1\n32461\t12005\tInlet beach\tFL\tBay County\tH1\n32462\t12005\tVernon\tFL\tBay County\tH1\n32401\t12005\tPanama city\tFL\tBay County\tH1\n32407\t12005\tPanama city beach\tFL\tBay County\tH1\n32410\t12005\tMexico beach\tFL\tBay County\tH1\n32413\t12005\tPanama city beach\tFL\tBay County\tH1\n32466\t12005\tYoungstown\tFL\tBay County\tH1\n32444\t12005\tLynn haven\tFL\tBay County\tH1\n32404\t12005\tPanama city\tFL\tBay County\tH1\n32402\t12005\tPanama city\tFL\tBay County\tH1\n32091\t12007\tStarke\tFL\tBradford County\tH1\n32609\t12007\tGainesville\tFL\tBradford County\tH1\n32058\t12007\tLawtey\tFL\tBradford County\tH1\n32656\t12007\tKeystone heights\tFL\tBradford County\tH1\n32622\t12007\tBrooker\tFL\tBradford County\tH1\n32666\t12007\tMelrose\tFL\tBradford County\tH1\n32042\t12007\tGraham\tFL\tBradford County\tH1\n32083\t12007\tRaiford\tFL\tBradford County\tH1\n32044\t12007\tHampton\tFL\tBradford County\tH1\n32054\t12007\tLake butler\tFL\tBradford County\tH1\n32026\t12007\tRaiford\tFL\tBradford County\tH1\n32901\t12009\tMelbourne\tFL\tBrevard County\tH1\n32908\t12009\tPalm bay\tFL\tBrevard County\tH1\n32952\t12009\tMerritt island\tFL\tBrevard County\tH1\n32905\t12009\tPalm bay\tFL\tBrevard County\tH1\n32920\t12009\tCape canaveral\tFL\tBrevard County\tH1\n32903\t12009\tIndialantic\tFL\tBrevard County\tH1\n32925\t12009\tPatrick afb\tFL\tBrevard County\tH1\n32953\t12009\tMerritt island\tFL\tBrevard County\tH1\n32941\t12009\tMelbourne\tFL\tBrevard County\tH1\n32923\t12009\tCocoa\tFL\tBrevard County\tH1\n32781\t12009\tTitusville\tFL\tBrevard County\tH1\n32909\t12009\tPalm bay\tFL\tBrevard County\tH1\n32950\t12009\tMalabar\tFL\tBrevard County\tH1\n32902\t12009\tMelbourne\tFL\tBrevard County\tH1\n32924\t12009\tCocoa\tFL\tBrevard County\tH1\n32906\t12009\tPalm bay\tFL\tBrevard County\tH1\n32959\t12009\tSharpes\tFL\tBrevard County\tH1\n32815\t12009\tOrlando\tFL\tBrevard County\tH1\n32899\t12009\tOrlando\tFL\tBrevard County\tH1\n32926\t12009\tCocoa\tFL\tBrevard County\tH1\n32783\t12009\tTitusville\tFL\tBrevard County\tH1\n32911\t12009\tPalm bay\tFL\tBrevard County\tH1\n32910\t12009\tPalm bay\tFL\tBrevard County\tH1\n32935\t12009\tMelbourne\tFL\tBrevard County\tH1\n32904\t12009\tMelbourne\tFL\tBrevard County\tH1\n32922\t12009\tCocoa\tFL\tBrevard County\tH1\n32937\t12009\tSatellite beach\tFL\tBrevard County\tH1\n32976\t12009\tSebastian\tFL\tBrevard County\tH1\n32932\t12009\tCocoa beach\tFL\tBrevard County\tH1\n32754\t12009\tMims\tFL\tBrevard County\tH1\n32780\t12009\tTitusville\tFL\tBrevard County\tH1\n32936\t12009\tMelbourne\tFL\tBrevard County\tH1\n32956\t12009\tRockledge\tFL\tBrevard County\tH1\n32775\t12009\tScottsmoor\tFL\tBrevard County\tH1\n32948\t12009\tFellsmere\tFL\tBrevard County\tH1\n32955\t12009\tRockledge\tFL\tBrevard County\tH1\n32931\t12009\tCocoa beach\tFL\tBrevard County\tH1\n32927\t12009\tCocoa\tFL\tBrevard County\tH1\n32934\t12009\tMelbourne\tFL\tBrevard County\tH1\n32912\t12009\tMelbourne\tFL\tBrevard County\tH1\n32940\t12009\tMelbourne\tFL\tBrevard County\tH1\n32951\t12009\tMelbourne beach\tFL\tBrevard County\tH1\n32907\t12009\tPalm bay\tFL\tBrevard County\tH1\n32949\t12009\tGrant\tFL\tBrevard County\tH1\n32796\t12009\tTitusville\tFL\tBrevard County\tH1\n32954\t12009\tMerritt island\tFL\tBrevard County\tH1\n33019\t12011\tHollywood\tFL\tBroward County\tH1\n33004\t12011\tDania\tFL\tBroward County\tH1\n33308\t12011\tFort lauderdale\tFL\tBroward County\tH1\n33062\t12011\tPompano beach\tFL\tBroward County\tH1\n33332\t12011\tFort lauderdale\tFL\tBroward County\tH1\n33329\t12011\tFort lauderdale\tFL\tBroward County\tH1\n33348\t12011\tFort lauderdale\tFL\tBroward County\tH1\n33024\t12011\tHollywood\tFL\tBroward County\tH1\n33021\t12011\tHollywood\tFL\tBroward County\tH1\n33022\t12011\tHollywood\tFL\tBroward County\tH1\n33076\t12011\tPompano beach\tFL\tBroward County\tH1\n33312\t12011\tFort lauderdale\tFL\tBroward County\tH1\n33323\t12011\tFort lauderdale\tFL\tBroward County\tH1\n33317\t12011\tFort lauderdale\tFL\tBroward County\tH1\n33306\t12011\tFort lauderdale\tFL\tBroward County\tH1\n33318\t12011\tFort lauderdale\tFL\tBroward County\tH1\n33325\t12011\tFort lauderdale\tFL\tBroward County\tH1\n33351\t12011\tFort lauderdale\tFL\tBroward County\tH1\n33307\t12011\tFort lauderdale\tFL\tBroward County\tH1\n33394\t12011\tFort lauderdale\tFL\tBroward County\tH1\n33388\t12011\tPlantation\tFL\tBroward County\tH1\n33009\t12011\tHallandale\tFL\tBroward County\tH1\n33071\t12011\tCoral springs\tFL\tBroward County\tH1\n33073\t12011\tPompano beach\tFL\tBroward County\tH1\n33319\t12011\tFort lauderdale\tFL\tBroward County\tH1\n33027\t12011\tHollywood\tFL\tBroward County\tH1\n33056\t12011\tMiami gardens\tFL\tBroward County\tH1\n33069\t12011\tPompano beach\tFL\tBroward County\tH1\n33327\t12011\tFort lauderdale\tFL\tBroward County\tH1\n33441\t12011\tDeerfield beach\tFL\tBroward County\tH1\n33061\t12011\tPompano beach\tFL\tBroward County\tH1\n33335\t12011\tFort lauderdale\tFL\tBroward County\tH1\n33310\t12011\tFort lauderdale\tFL\tBroward County\tH1\n33020\t12011\tHollywood\tFL\tBroward County\tH1\n33023\t12011\tHollywood\tFL\tBroward County\tH1\n33008\t12011\tHallandale\tFL\tBroward County\tH1\n33309\t12011\tFort lauderdale\tFL\tBroward County\tH1\n33301\t12011\tFort lauderdale\tFL\tBroward County\tH1\n33063\t12011\tPompano beach\tFL\tBroward County\tH1\n33067\t12011\tPompano beach\tFL\tBroward County\tH1\n33331\t12011\tFort lauderdale\tFL\tBroward County\tH1\n33330\t12011\tFort lauderdale\tFL\tBroward County\tH1\n33075\t12011\tCoral springs\tFL\tBroward County\tH1\n33081\t12011\tHollywood\tFL\tBroward County\tH1\n33083\t12011\tHollywood\tFL\tBroward County\tH1\n33179\t12011\tMiami\tFL\tBroward County\tH1\n33060\t12011\tPompano beach\tFL\tBroward County\tH1\n33029\t12011\tHollywood\tFL\tBroward County\tH1\n33065\t12011\tCoral springs\tFL\tBroward County\tH1\n33328\t12011\tFort lauderdale\tFL\tBroward County\tH1\n33334\t12011\tFort lauderdale\tFL\tBroward County\tH1\n33359\t12011\tFort lauderdale\tFL\tBroward County\tH1\n33084\t12011\tHollywood\tFL\tBroward County\tH1\n33093\t12011\tMargate\tFL\tBroward County\tH1\n33443\t12011\tDeerfield beach\tFL\tBroward County\tH1\n33077\t12011\tPompano beach\tFL\tBroward County\tH1\n33346\t12011\tFort lauderdale\tFL\tBroward County\tH1\n33018\t12011\tHialeah\tFL\tBroward County\tH1\n33025\t12011\tHollywood\tFL\tBroward County\tH1\n33314\t12011\tFort lauderdale\tFL\tBroward County\tH1\n33322\t12011\tFort lauderdale\tFL\tBroward County\tH1\n33026\t12011\tHollywood\tFL\tBroward County\tH1\n33324\t12011\tFort lauderdale\tFL\tBroward County\tH1\n33326\t12011\tFort lauderdale\tFL\tBroward County\tH1\n33345\t12011\tFort lauderdale\tFL\tBroward County\tH1\n33339\t12011\tFort lauderdale\tFL\tBroward County\tH1\n33097\t12011\tCoconut creek\tFL\tBroward County\tH1\n33304\t12011\tFort lauderdale\tFL\tBroward County\tH1\n33305\t12011\tFort lauderdale\tFL\tBroward County\tH1\n33316\t12011\tFort lauderdale\tFL\tBroward County\tH1\n33064\t12011\tPompano beach\tFL\tBroward County\tH1\n33338\t12011\tFort lauderdale\tFL\tBroward County\tH1\n33442\t12011\tDeerfield beach\tFL\tBroward County\tH1\n33320\t12011\tFort lauderdale\tFL\tBroward County\tH1\n33074\t12011\tPompano beach\tFL\tBroward County\tH1\n33082\t12011\tPembroke pines\tFL\tBroward County\tH1\n33311\t12011\tFort lauderdale\tFL\tBroward County\tH1\n33313\t12011\tFort lauderdale\tFL\tBroward County\tH1\n33321\t12011\tFort lauderdale\tFL\tBroward County\tH1\n33315\t12011\tFort lauderdale\tFL\tBroward County\tH1\n33028\t12011\tPembroke pines\tFL\tBroward County\tH1\n33068\t12011\tPompano beach\tFL\tBroward County\tH1\n33066\t12011\tPompano beach\tFL\tBroward County\tH1\n33355\t12011\tFort lauderdale\tFL\tBroward County\tH1\n33302\t12011\tFort lauderdale\tFL\tBroward County\tH1\n32420\t12013\tAlford\tFL\tCalhoun County\tH1\n32438\t12013\tFountain\tFL\tCalhoun County\tH1\n32465\t12013\tWewahitchka\tFL\tCalhoun County\tH1\n32430\t12013\tClarksville\tFL\tCalhoun County\tH1\n32424\t12013\tBlountstown\tFL\tCalhoun County\tH1\n32466\t12013\tYoungstown\tFL\tCalhoun County\tH1\n32421\t12013\t
